vi "Actor Core.vi"(8 "error in (no error)":errorcluster, 11 "Child Actor in":refnum<class "Child Actor.lvclass">) -> (0 "error out":errorcluster, 3 "Child Actor out":refnum<class "Child Actor.lvclass">)   [LabVIEW 2015, in "Child Actor.lvclass"]
uses:
  Child Actor.lvclass
  State/Parent Actor.lvclass/Parent Actor.ctl
  State/Parent Actor.lvclass
  Parent Message/Parent Message.lvclass
  Toggle/Toggle.lvclass
panel:
  in  "Dirrection control":enum16{"Forward", "Reverse"}(ring)
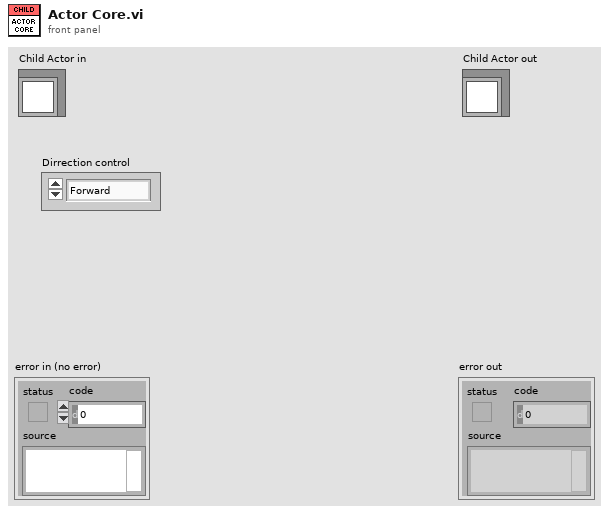
[diagram p1: front panel]
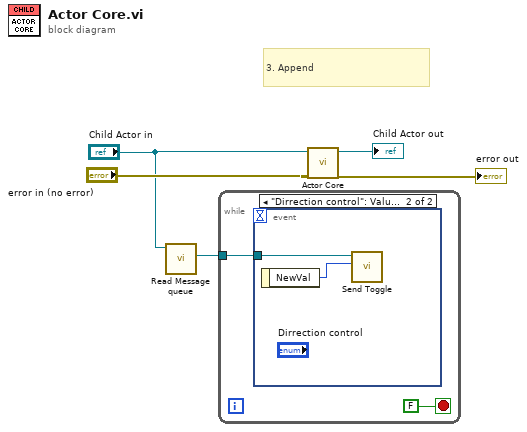
[diagram p0: block diagram]
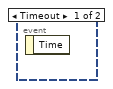
[diagram p2: hidden frame]
diagram:
  # "3. Append"
  n1 = call "Read Message queue.vi"("Parent Actor in"="Child Actor in") -> ("Message queue"=w1:refnum<queue>)  [unwired: 8 in, 2 out]
  n2 = while {
    tunnel: w1 -> [w7]
    stop <- FALSE stop-if-true
    n3 = event shown="[1] \"Dirrection control\": Value Change" {
      selector: _ -> [_ _]
      dyn-events: _ -> [_ _]
      timeout: _ -> [_ _]
      tunnel: w7 -> [_ w9]
      event Timeout {
        n4 = event-data() -> ()  [unwired: 1 in, 1 out]
      }
      event "Dirrection control": Value Change {
        n5 = event-data() -> ("NewVal"=w8:enum16{"Forward", "Reverse"})  [unwired: 1 in]
        n6 = call "Send Toggle.vi"("Dirrection"=w8, "Message queue"=w9) -> ()  [unwired: 9 in, 1 out]
      }
    }
  }
  n7 = call-parent "Actor Core.vi"("error in (no error)"="error in (no error)", "Parent Actor in"="Child Actor in") -> ("error out"=→"error out":errorcluster, "Parent Actor out"=→"Child Actor out":refnum<class "Child Actor.lvclass">)  [unwired: 8 in]
